vi "ExSub4ROI.vi"(2 "error in (no error)":errorcluster, 3 "Camera Handle":u32) -> (0 "error out":errorcluster, 1 "Camera Handle":u32)   [LabVIEW 2010]
panel:
  # "ExSub4ROI:\nThis is a Sub-VI that defines 4 ROIs, it defines them \nso that the 4 corners of the CCD chip are displayed."
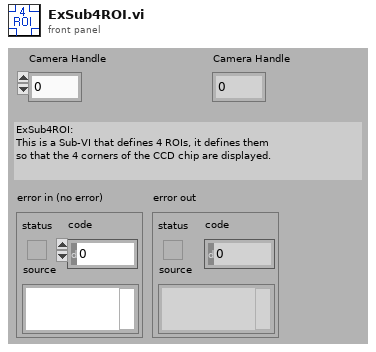
[diagram p1: front panel]
types:
  T1 = cluster{i32, "Xdim":u32, i32, i32, "Ydim":u32, i32}
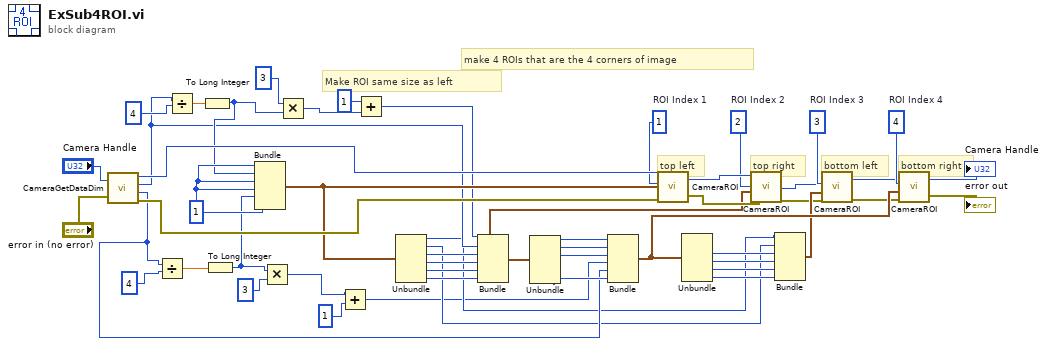
[diagram p0: block diagram]
diagram:
  w7 = 3  # ROI Index 3
  w36 = 4  # ROI Index 4
  w44 = 2  # ROI Index 2
  w47 = 1  # ROI Index 1
  w35 = 1
  # "top left"
  # "bottom left"
  # "Make ROI same size as left"
  # "bottom right"
  # "top right"
  # "make 4 ROIs that are the 4 corners of image"
  n1 = call <userlib>:"CameraGetDataDim.vi"("Camera Handle"="Camera Handle", "error in"="error in (no error)") -> ("Camera Handle"=w50:u32, "Xdim"=w27:u32, "Ydim"=w22:u32, "error out"=w48:errorcluster)
  n2 = Divide(x=w22, y=4) -> (x/y=w32:dbl)
  n3 = Divide(x=w27, y=4) -> (x/y=w33:dbl)
  n4 = To Long Integer(number=w33) -> (32bit integer=w30:i32)
  n5 = To Long Integer(number=w32) -> (32bit integer=w26:i32)
  n6 = Bundle(w35, w30, w35, w35, w26, w35) -> (w43:cluster{i32, i32, i32, i32, i32, i32})  [unwired: 1 in]
  n7 = Multiply(x=w26, y=3) -> (x*y=w10:i32)
  n8 = Multiply(x=3, y=w30) -> (x*y=w13:i32)
  n9 = Add(x=w10, y=1) -> (x+y=w8:i32)
  n10 = Add(x=1, y=w13) -> (x+y=w11:i32)
  n11 = Unbundle(w43) -> (w15:i32, w16:i32, w42:i32, w29:i32, w28:i32, w41:i32)
  n12 = Bundle(w11, "Xdim"=w27, w42, w29, w28, w41) -> (w39:cluster{i32, "Xdim":u32, i32, i32, i32, i32})  [unwired: 1 in]
  n13 = Unbundle(w39) -> (w24:i32, "Xdim"=w23:u32, w38:i32, w37:i32)  [unwired: 2 out]
  n14 = Bundle(w24, "Xdim"=w23, w38, w8, "Ydim"=w22, w37) -> (w21:T1)  [unwired: 1 in]
  n15 = call <userlib>:"CameraROI.vi"("error in"=w48, "ROI Params"=w43, "ROI Index"=w47, "Camera Handle"=w50) -> ("error out"=w40:errorcluster, "Camera Handle"=w45:u32)
  n16 = Unbundle(w21) -> (w17:i32, w18:i32, "Ydim"=w19:u32, w20:i32)  [unwired: 2 out]
  n17 = call <userlib>:"CameraROI.vi"("error in"=w40, "ROI Params"=w39, "ROI Index"=w44, "Camera Handle"=w45) -> ("error out"=w1:errorcluster, "Camera Handle"=w6:u32)
  n18 = Bundle(w15, w16, w17, w18, "Ydim"=w19, w20) -> (w14:cluster{i32, i32, i32, i32, "Ydim":u32, i32})  [unwired: 1 in]
  n19 = call <userlib>:"CameraROI.vi"("error in"=w1, "ROI Params"=w14, "ROI Index"=w7, "Camera Handle"=w6) -> ("error out"=w4:errorcluster, "Camera Handle"=w5:u32)
  n20 = call <userlib>:"CameraROI.vi"("error in"=w4, "ROI Params"=w21, "ROI Index"=w36, "Camera Handle"=w5) -> ("error out"=→"error out":errorcluster, "Camera Handle"=→"Camera Handle":u32)
